vi "create.vi"(8 "error in":errorcluster) -> (0 "error out":errorcluster, 3 "midi-file-events":refnum<class "midi-file-events.lvclass">)   [LabVIEW 2020, in "midi-file-events.lvclass"]
uses:
  midi-file-events.lvclass
  midi-file-event/midi-file-event.lvclass
  privatedata.ctl
  midi-file-event.midi/midi-file-event.midi.lvclass
  midi-file-events.lvclass/midi-file-events.ctl
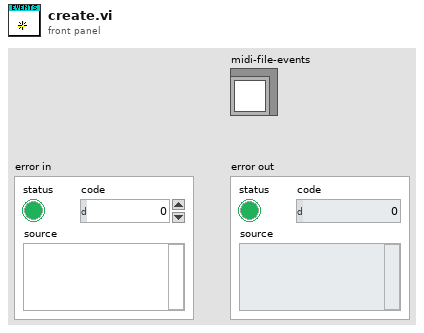
[diagram p1: front panel]
types:
  T1 = typedef "midi-file-events.lvclass/privatedata.ctl" = cluster{"ticks per quarter note (division)":i16, "Tempo Map":map{dbl, dbl}, "Track data by Track number":map{i32, map{dbl, set{refnum<class "midi-file-event.midi.lvclass">}}}}
  T2 = map{i32, refnum<class "midi-file-event.lvclass">[]}
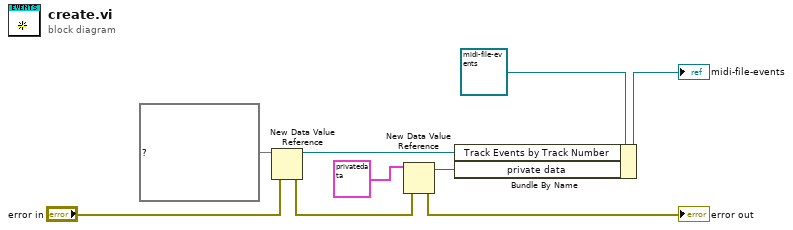
[diagram p0: block diagram]
diagram:
  n1 = New Data Value Reference(data value=T2 {} ("Track Events by Track Number"), error in="error in") -> (data value reference=w6:refnum<data-value>, error out=w1:errorcluster)
  n2 = New Data Value Reference(data value=T1 {"ticks per quarter note (division)"=0, "Tempo Map"={}, "Track data by Track number"={}} ("private data"), error in=w1) -> (data value reference=w4:refnum<data-value>, error out=→"error out":errorcluster)
  n3 = Bundle By Name(cluster=refnum<class "midi-file-events.lvclass"> refnum ("midi-file-events"), "Track Events by Track Number"=w6, "private data"=w4) -> (→"midi-file-events":refnum<class "midi-file-events.lvclass">)
